vi "Event Actor.vi"(4 "Queue Nested":map{string, refnum<data-value>}(c390), 6 "Queue Self":map{string, refnum<data-value>}(c390), 8 "Queue Caller":map{string, refnum<data-value>}(c390), 9 "Queue of Event Self":refnum<queue>, 10 "Event Self Alias":string, 11 "Event jettl":refnum<class "Event jettl.lvclass">) -> ()   [LabVIEW 2021, in "jettl.lvlib" / "Base Event jettl.lvlib" / "Base Event jettl.lvclass"]
uses:
  Base Event jettl.lvclass
  Event jettl/Event jettl.lvclass
  Msg Strategy/Msg Strategy/Msg Strategy.lvclass
  C:/git/jettl/src/jettl/jettl/Event jettl/Event jettl.lvclass
  Msg Strategy/Event Last Ack/Event Last Ack Msg Strategy/Event Last Ack Msg Strategy.lvclass
  C:/git/jettl/src/jettl/Msg Strategy/Msg Strategy/Msg Strategy.lvclass
  jettl.lvlib
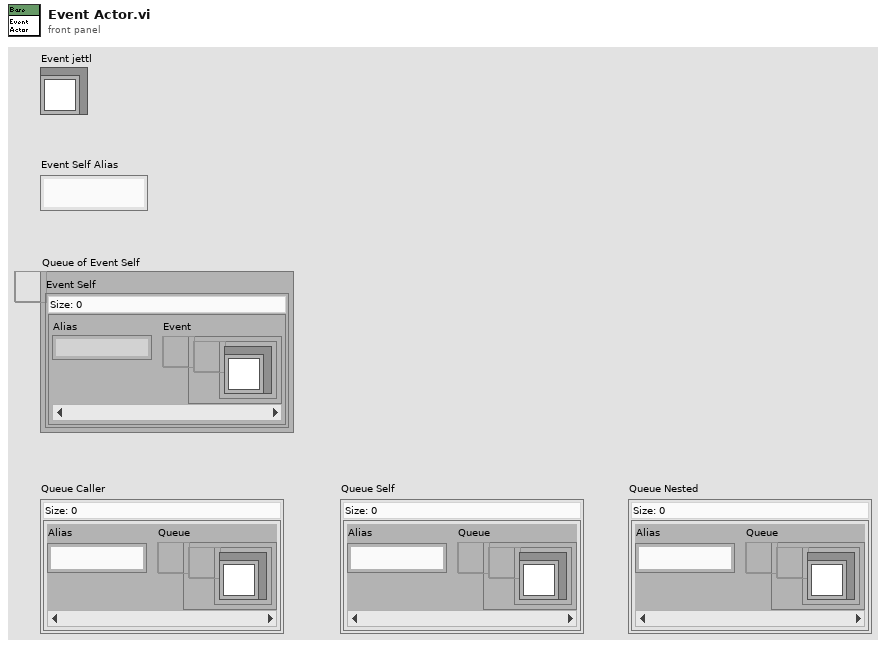
[diagram p1: front panel]
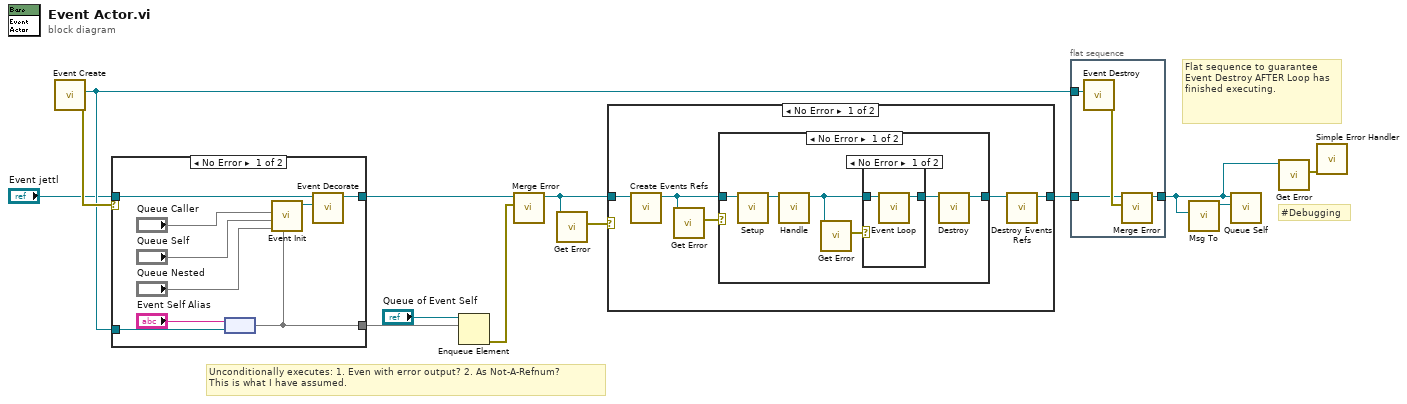
[diagram p0: block diagram]
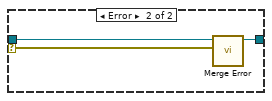
[diagram p2: hidden frame]
diagram:
  # "Flat sequence to guarantee Event Destroy AFTER Loop has finished executing."
  # "Unconditionally executes: 1. Even with error output? 2. As Not-A-Refnum?\nThis is what I have assumed."
  # "#Debugging"
  n1 = call "Event Create.vi"() -> ("error out"=w7:errorcluster, "Event"=w6:refnum<data-value>)  [unwired: 10 in]
  n2 = case shown="No Error" w7 {
    selector: w7 -> [_ w24]
    tunnel: [w14 w25] -> w11
    tunnel: "Event jettl" -> [w21 w23]
    tunnel: w6 -> [w22 _]
    tunnel: [w20 _] -> w10
    frame No Error {
      n3 = node("Event Self Alias", w22) -> (w20:map{string, refnum<data-value>})
      n4 = call "Event Init.vi"("Event Self"=w20, "Queue Nested"="Queue Nested", "Queue Self"="Queue Self", "Queue Caller"="Queue Caller") -> ("Base Event jettl out"=w15:refnum<class "Base Event jettl.lvclass">)  [unwired: 7 in]
      n5 = call-dynamic "Event Decorate.vi"("Event jettl"=w15, "Event jettl in"=w21) -> ("Event jettl out"=w14:refnum<class "Event jettl.lvclass">)  [unwired: 9 in]
    }
    frame Error {
      n6 = call-dynamic "Merge Error.vi"("Error"=w24, "jettl in"=w23) -> ("jettl out"=w25:refnum<class "Event jettl.lvclass">)  [unwired: 9 in]
    }
  }
  n7 = Enqueue Element(queue="Queue of Event Self", element=w10) -> (error out=w12:errorcluster)  [unwired: 2 in, 2 out]
  n8 = call-dynamic "Merge Error.vi"("Error"=w12, "jettl in"=w11) -> ("jettl out"=w13:refnum<class "Event jettl.lvclass">)  [unwired: 9 in]
  n9 = call-dynamic "Get Error.vi"("jettl in"=w13) -> ("Error"=w9:errorcluster)  [unwired: 10 in]
  n10 = case shown="No Error" w9 {
    tunnel: w13 -> [w30 w41]
    tunnel: [w26 w41] -> w8
    frame No Error {
      n11 = call-dynamic "Create Events Refs.vi"("Event jettl in"=w30) -> ("Event jettl out"=w28:refnum<class "Event jettl.lvclass">)  [unwired: 10 in]
      n12 = call-dynamic "Get Error.vi"("jettl in"=w28) -> ("Error"=w29:errorcluster)  [unwired: 10 in]
      n13 = case shown="No Error" w29 {
        tunnel: w28 -> [w36 w40]
        tunnel: [w31 w40] -> w27
        frame No Error {
          n14 = call-dynamic "Setup.vi"("Setup in"=w36) -> ("Setup out"=w35:refnum<class "Event jettl.lvclass">)  [unwired: 10 in]
          n15 = call-dynamic "Handle.vi"("jettl in"=w35) -> ("jettl out"=w34:refnum<class "Event jettl.lvclass">)  [unwired: 9 in, 1 out]
          n16 = call-dynamic "Get Error.vi"("jettl in"=w34) -> ("Error"=w33:errorcluster)  [unwired: 10 in]
          n17 = case shown="No Error" w33 {
            tunnel: [w37 w39] -> w32
            tunnel: w34 -> [w38 w39]
            frame No Error {
              n18 = call-dynamic "Event Loop.vi"("Event jettl in"=w38) -> ("Event jettl out"=w37:refnum<class "Event jettl.lvclass">)  [unwired: 10 in]
            }
            frame Error {
            }
          }
          n19 = call-dynamic "Destroy.vi"("jettl in"=w32) -> ("jettl out"=w31:refnum<class "Event jettl.lvclass">)  [unwired: 10 in]
        }
        frame Error {
        }
      }
      n20 = call-dynamic "Destroy Events Refs.vi"("Event jettl in"=w27) -> ("Event jettl out"=w26:refnum<class "Event jettl.lvclass">)  [unwired: 10 in]
    }
    frame Error {
    }
  }
  n21 = flat-sequence {
    tunnel: w6 -> [w44]
    tunnel: [w45] -> w1
    tunnel: w8 -> [w42]
    frame #0 {
      n22 = call "Event Destroy.vi"("Event"=w44) -> ("error out"=w43:errorcluster)  [unwired: 10 in]
      n23 = call-dynamic "Merge Error.vi"("Error"=w43, "jettl in"=w42) -> ("jettl out"=w45:refnum<class "Event jettl.lvclass">)  [unwired: 9 in]
    }
  }
  n24 = call "Msg To.vi"("Event jettl"=w1) -> ("Event Last Ack Msg out"=w3:refnum<class "Event Last Ack Msg Strategy.lvclass">)  [unwired: 10 in]
  n25 = call-dynamic "Queue Self.vi"("Msg Strategy"=w3, "jettl in"=w1) -> ()  [unwired: 9 in, 1 out]
  n26 = call-dynamic "Get Error.vi"("jettl in"=w1) -> ("Error"=w2:errorcluster)  [unwired: 10 in]
  n27 = call <vilib>:"Simple Error Handler.vi"("error in (no error)"=w2) -> ()  [unwired: 4 in, 5 out]
